vi "PPG_ABC.load ABC.vi"(0 "i ref in":refnum<vi>, 1 "PGData":T1, 2 "patternGroup":i32, 3 "ms timeout [ms]":i32=10000, 5 "error in (no error)":errorcluster) -> (14 "i ref out":refnum<vi>, 17 "timed out":bool, 19 "error out":errorcluster)   [LabVIEW 2014, in "PPG_ABC.lvlib"]
doc: "Loads a pattern given in a dedicated format."
uses:
  PPG_ABC.lvlib
  PPG_ABC.PG_dataType.ctl
  NI_FPGA_PPG/NI_FPGA_PPG.lvlib
  CS_Core/CSSystem/CoreLib/CoreLib.lvlib
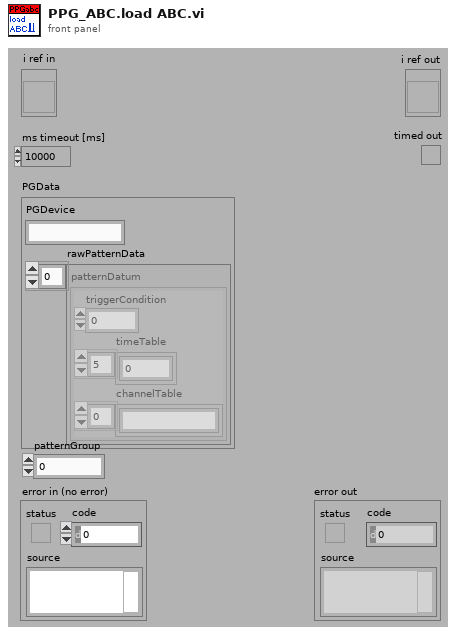
[diagram p1: front panel]
types:
  T1 = typedef "PPG_ABC.lvlib/PPG_ABC.PG_dataType.ctl" = cluster{"PGDevice":string, "rawPatternData":cluster{"triggerCondition":i32, "timeTable":dbl[], "channelTable":string[]}[]}
  T2 = typedef "PPG_ABC.lvlib/PPG_ABC.i attribute.ctl" = cluster{"patternGroups":T1[], "defaultLetter":string, "defaultPatternGroup":i32, "PGRunning":T3, "PGRunningID":i32, "pgStarting":T4}
  T3 = typedef "PPG_ABC.lvlib/PPG_ABC.PG_Running.ctl" = i32
  T4 = typedef "Semaphore RefNum" = refnum<k1>
  T5 = cluster{"Mem 0":u8, "Mem 1":u32, "Mem 2":u32, "Mem 3":u32}[]
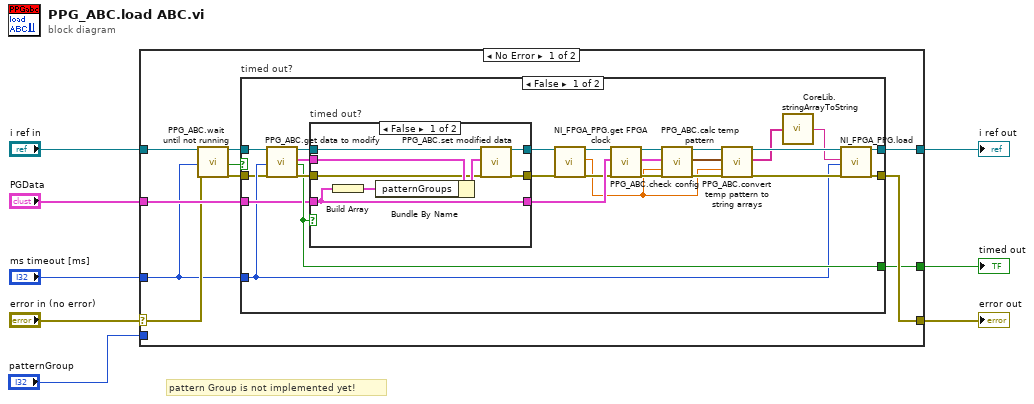
[diagram p0: block diagram]
diagram:
  # "pattern Group is not implemented yet!"
  n1 = case shown="No Error" "error in (no error)" {
    selector: "error in (no error)" -> [w13 w60]
    tunnel: [w17 w60] -> w7
    tunnel: "i ref in" -> [w14 w59]
    tunnel: [w18 w59] -> w5
    tunnel: "PGData" -> [w15 _]
    tunnel: "ms timeout [ms]" -> [w12 _]
    tunnel: [w16 _] -> w2
    tunnel: "patternGroup" -> [_ _]
    frame No Error {
      n2 = call "PPG_ABC.wait until not running.vi"("i ref in"=w14, "ms timeout (10000)"=w12, "error in (no error)"=w13) -> ("i ref out"=w10:refnum<vi>, "timed out"=w9:bool, "error out"=w11:errorcluster)  [unwired: 14 in]
      n3 = case "timed out?" shown="False" w9 {
        selector: w9 -> [_ w56]
        tunnel: [w44 w58] -> w18
        tunnel: [w43 w57] -> w17
        tunnel: [w40 w56] -> w16
        tunnel: w15 -> [w36 _]
        tunnel: w12 -> [w29 _]
        tunnel: w11 -> [w28 w57]
        tunnel: w10 -> [w27 w58]
        frame False {
          n4 = call "PPG_ABC.get data to modify.vi"("i ref in"=w27, "ms timeout (10000)"=w29, "error in (no error)"=w28) -> ("i ref out"=w42:refnum<vi>, "i attribute"=w37:T2, "timed out"=w40:bool, "error out"=w41:errorcluster)  [unwired: 13 in]
          n5 = case "timed out?" shown="False" w40 {
            tunnel: [w51 w54] -> w20
            tunnel: [w52 w55] -> w23
            tunnel: w42 -> [w46 w55]
            tunnel: w41 -> [w47 w54]
            tunnel: w37 -> [w50 _]
            tunnel: w36 -> [w48 w53]
            tunnel: [w48 w53] -> w35
            frame False {
              n6 = Build Array(w48) -> (w45:T1[])
              n7 = Bundle By Name(cluster=w50, "patternGroups"=w45) -> (w49:T2)
              n8 = call "PPG_ABC.set modified data.vi"("i ref in"=w46, "i attribute"=w49, "error in (no error)"=w47) -> ("i ref out"=w52:refnum<vi>, "error out"=w51:errorcluster)  [unwired: 15 in]
            }
            frame True {
            }
          }
          n9 = call "NI_FPGA_PPG.get FPGA clock.vi"("i ref in"=w23, "error in (no error)"=w20) -> ("i ref out"=w22:refnum<vi>, "clockRate [ticks/us]"=w19:dbl, "error out"=w21:errorcluster)  [unwired: 15 in]
          n10 = call "PPG_ABC.check config.vi"("i ref in"=w22, "PGData"=w35, "error in (no error)"=w21) -> ("i ref out"=w25:refnum<vi>, "PGData out"=w26:T1, "error out"=w24:errorcluster)  [unwired: 14 in]
          n11 = call "PPG_ABC.calc temp pattern.vi"("i ref in"=w25, "PGData"=w26, "clockRate [ticks/us]"=w19, "error in (no error)"=w24) -> ("i ref out"=w38:refnum<vi>, "patternDefs"=w34:T5, "error out"=w39:errorcluster)  [unwired: 13 in]
          n12 = call "PPG_ABC.convert temp pattern to string arrays.vi"("i ref in"=w38, "patternDefs"=w34, "clockRate [ticks/us]"=w19, "error in (no error)"=w39) -> ("i ref out"=w33:refnum<vi>, "patternArray"=w32:string[], "error out"=w31:errorcluster)  [unwired: 13 in]
          n13 = call "CoreLib.stringArrayToString.vi"("Array"=w32) -> ("String"=w30:string)
          n14 = call "NI_FPGA_PPG.load.vi"("i ref in"=w33, "cmd_data_string"=w30, "ms timeout (10000)"=w29, "error in (no error)"=w31) -> ("i ref out"=w44:refnum<vi>, "error out"=w43:errorcluster)  [unwired: 13 in, 1 out]
        }
        frame True {
        }
      }
    }
    frame Error {
    }
  }
  "error out" <- w7
  "i ref out" <- w5
  "timed out" <- w2
